vi "UMLEditor reversedEngineeringRecursiveInheritInfo.vi"(1 "localIn":T1 {"block"."bounds"."height" format="%.2f"; "block"."bounds"."width" format="%.2f"; "block"."bounds"."y" format="%.2f"; "block"."bounds"."x" format="%.2f"; "bounds"."height" format="%.2f"; "bounds"."width" format="%.2f"; "bounds"."y" format="%.2f"; "bounds"."x" format="%.2f"}, 2 "nodeIndex":i32, 3 "widthGap":i32=50, 4 "heightGap":i32=50, 5 "error in (no error)":errorcluster, 7 "allInheritorIn":i32[](array[numeric])) -> (9 "BlockHeight":i32, 11 "myHeight":i32, 13 "myWidth":i32, 14 "inheritorFound":bool, 15 "width":i32, 16 "myInheritor":i32[](array[numeric]), 17 "allInheritor":i32[](array[numeric]), 18 "myInheritorWidth":i32[](array[numeric]), 19 "error out":errorcluster)   [LabVIEW 2012]
doc: "Gets current diagram values"
uses:
  <resource>/Framework/Providers/Open_GDS/UML/UMLEditor/UMLEditor RevEngLocalvarType.ctl
  <resource>/Framework/Providers/Open_GDS/UML/Graph_class/Graph.lvclass
  <resource>/Framework/Providers/Open_GDS/UML/Graphics_class/Graphics.lvclass
  <resource>/Framework/Providers/Open_GDS/UML/Grid_class/Grid.lvclass
  <resource>/Framework/Providers/Open_GDS/UML/ClassNode_class/ClassNode.lvclass
  <resource>/Framework/Providers/Open_GDS/UML/AbstractEdge_class/AbstractEdge.lvclass
  <resource>/Framework/Providers/Open_GDS/UML/AbstractNode_class/AbstractNode.lvclass
  <resource>/Framework/Providers/Open_GDS/UML/ReversedEngineering/ReversedEngineering ClassInfoType.ctl
  <resource>/Framework/Providers/Open_GDS/UML/UMLEditor/UMLEditor_VisibilityType.ctl
  <resource>/Framework/Providers/Open_GDS/UML/ReversedEngineering/ReversedEngineering AttributeInfoType.ctl
  <resource>/Framework/Providers/Open_GDS/ClassProviders/Common/CommonVIs/CommonVIs_AttributeDataType.ctl
  <resource>/Framework/Providers/Open_GDS/UML/ReversedEngineering/ReversedEngineering_ClassDependencyDetailsType.ctl
  <resource>/Framework/Providers/Open_GDS/ClassProviders/Common/ScriptingFunctions/SubVIs/Scripting_ViDependencyType.ctl
  <resource>/Framework/Providers/Open_GDS/UML/General/Rectangle/Rectangle Rectangle2D.ctl
  <resource>/Framework/Providers/Open_GDS/UML/ReversedEngineering/ReversedEngineering TypeDefType.ctl
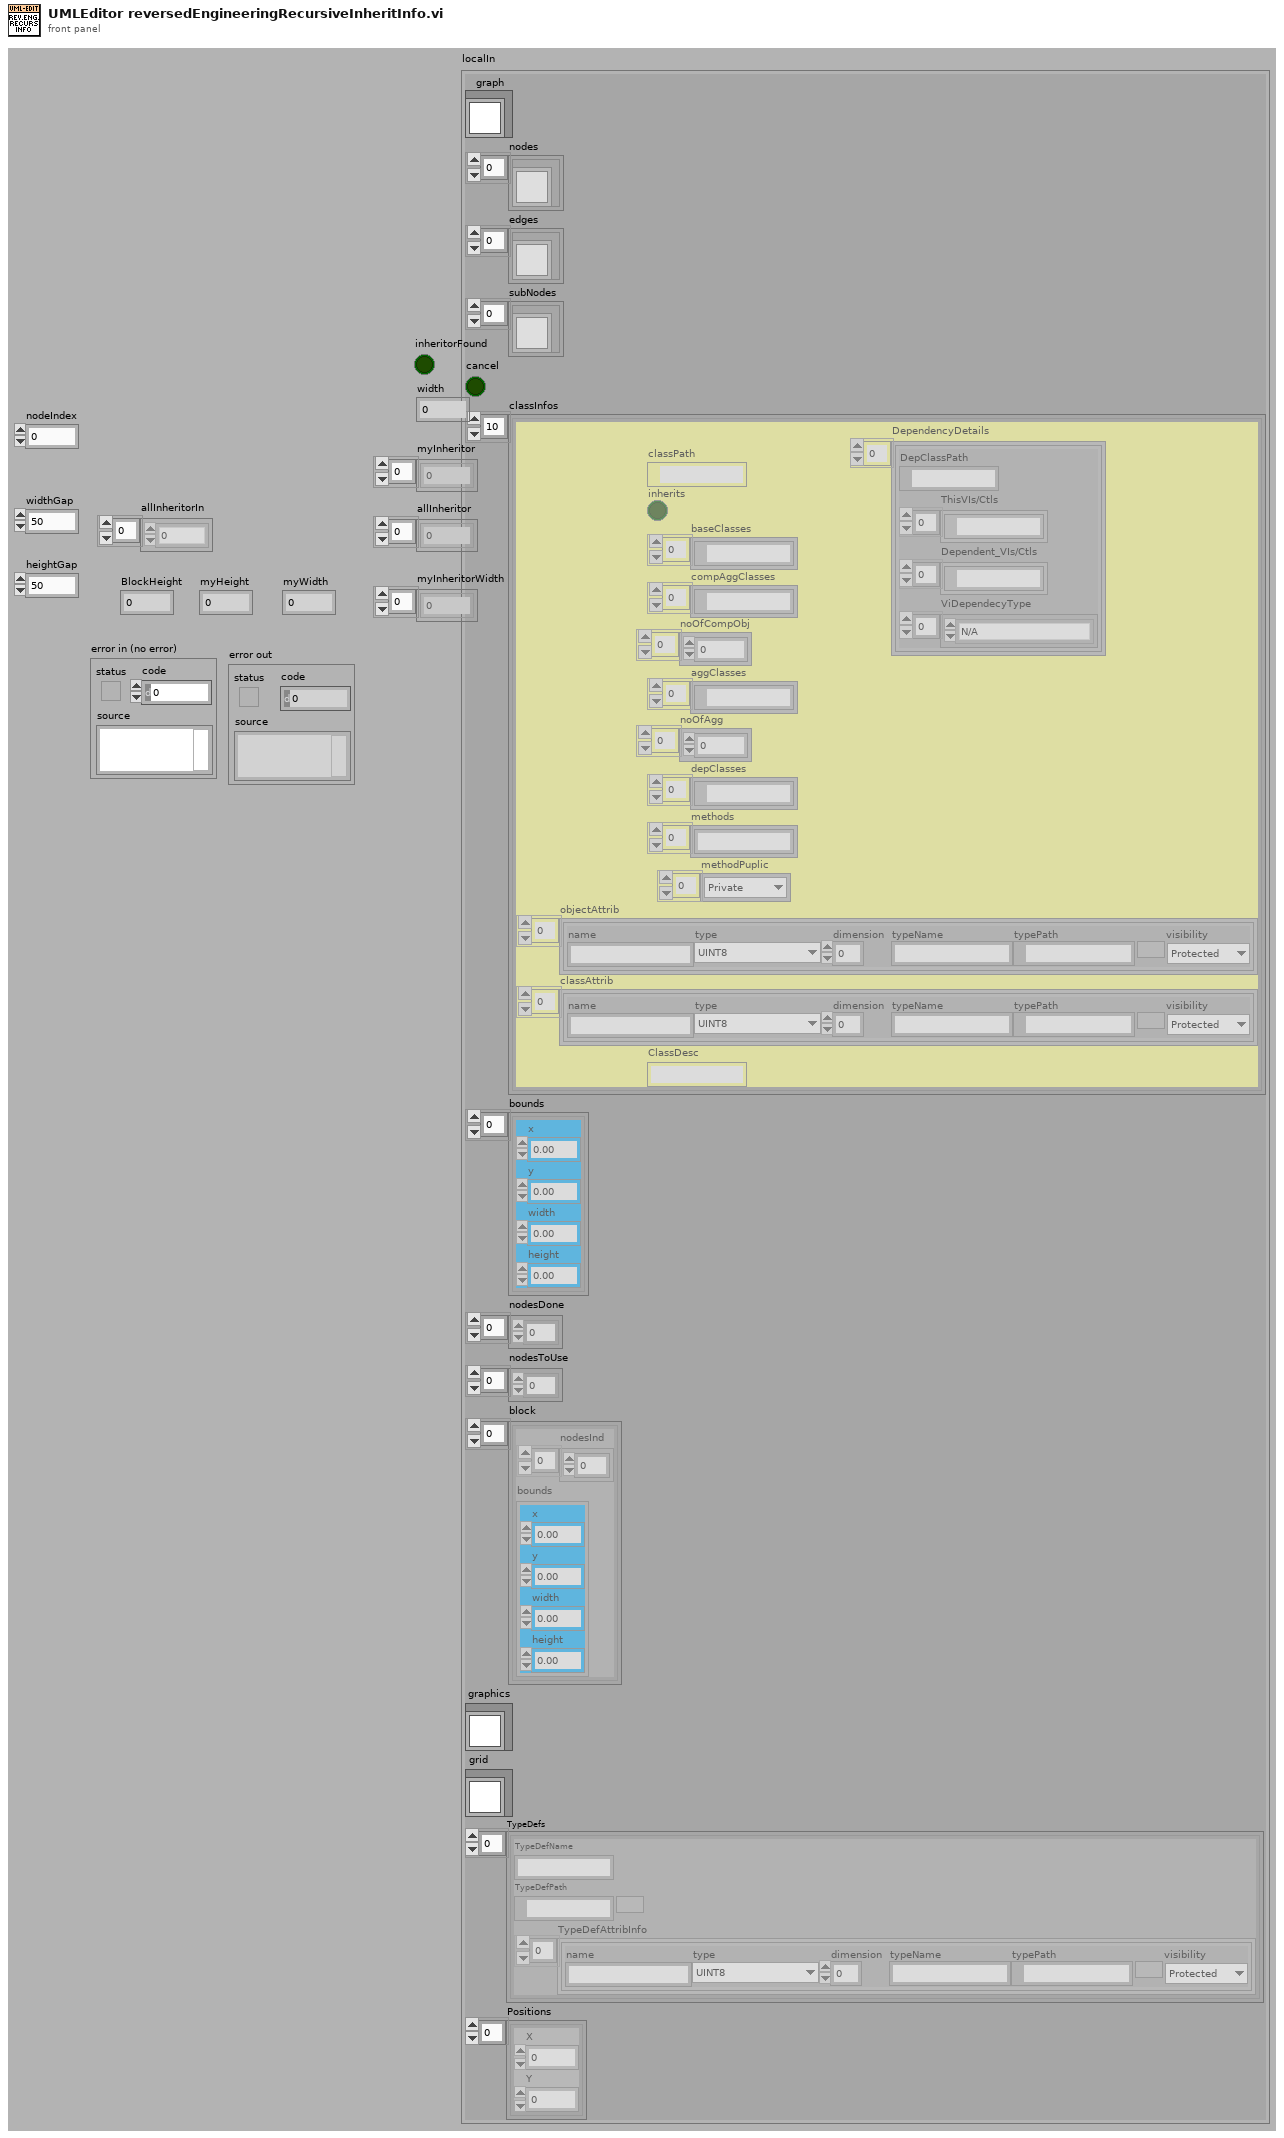
[diagram p1: front panel]
types:
  T1 = typedef "UMLEditor RevEngLocalvarType.ctl" = cluster{"graph":refnum<class "Graph.lvclass">, "nodes":refnum<class "ClassNode.lvclass">[], "edges":refnum<class "AbstractEdge.lvclass">[], "subNodes":refnum<class "AbstractNode.lvclass">[], "cancel":bool, "classInfos":T2[], "bounds":T8[], "nodesDone":i32[], "nodesToUse":i32[], "block":cluster{"nodesInd":i32[], "bounds":T8}[], "graphics":refnum<class "Graphics.lvclass">, "grid":refnum<class "Grid.lvclass">, "TypeDefs":T9[], "Positions":cluster{"X":i32, "Y":i32}[]}
  T2 = typedef "ReversedEngineering ClassInfoType.ctl" = cluster{"classPath":path, "inherits":bool, "baseClasses":path[], "compAggClasses":path[], "noOfCompObj":i32[], "aggClasses":path[], "noOfAgg":i32[], "depClasses":path[], "methods":string[], "methodPuplic":T3[], "objectAttrib":T4[], "classAttrib":T4[], "ClassDesc":string, "DependencyDetails":T6[]}
  T3 = typedef "UMLEditor_VisibilityType.ctl" = enum16{"Public", "Private", "Protected"}
  T4 = typedef "ReversedEngineering AttributeInfoType.ctl" = cluster{"name":string, "type":T5, "dimension":i32, "typeName":string, "typePath":path, "visibility":T3}
  T5 = typedef "CommonVIs_AttributeDataType.ctl" = enum16{"UINT8", "INT8", "UINT16", "INT16", "UINT32", "INT32", "UINT64", "INT64", "SGL", "DBL", "EXT", "CSG", "CDB", "CXT", "TimeStamp", "STRING", "PATH", "BOOL", "ENUM", "RefNum", "VIRefNum", "LabVIEW Class", "Cluster", "Variant", "TypeDef", "Waveform", "LabVIEW Object", "Other", "void"}
  T6 = typedef "ReversedEngineering_ClassDependencyDetailsType.ctl" = cluster{"DepClassPath":path, "ThisVIs/Ctls":path[], "Dependent_VIs/Ctls":path[], "ViDependecyType":T7[]}
  T7 = typedef "Scripting_ViDependencyType.ctl" = enum16{"N/A", "Launches"}
  T8 = typedef "Rectangle Rectangle2D.ctl" = cluster{"x":dbl, "y":dbl, "width":dbl, "height":dbl}
  T9 = typedef "ReversedEngineering TypeDefType.ctl" = cluster{"TypeDefName":string, "TypeDefPath":path, "TypeDefAttribInfo":T4[]}
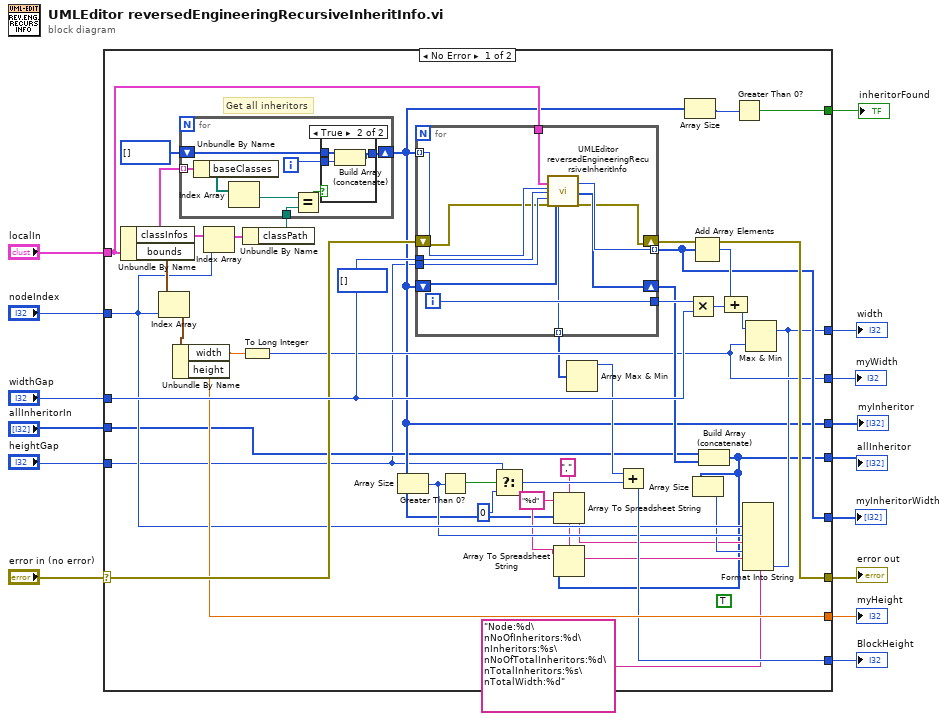
[diagram p0: block diagram]
diagram:
  n1 = case shown="No Error" "error in (no error)" {
    selector: "error in (no error)" -> [w43 w79]
    tunnel: [w42 w79] -> w14
    tunnel: "localIn" -> [w49 _]
    tunnel: "nodeIndex" -> [w26 _]
    tunnel: "widthGap" -> [w47 _]
    tunnel: [w27 _] -> w10
    tunnel: [w19 _] -> w9
    tunnel: [w18 _] -> w8
    tunnel: [w39 _] -> w7
    tunnel: [w38 _] -> w6
    tunnel: [w36 _] -> w5
    tunnel: [w35 _] -> w4
    tunnel: "heightGap" -> [w16 _]
    tunnel: [w31 _] -> w2
    tunnel: "allInheritorIn" -> [w17 _]
    frame No Error {
      (unwired) i32[] []
      w22 = "%d" ("format string")
      (unwired) TRUE ("convert eol? (no:F)")
      w21 = "," ("delimiter (Tab)")
      # "Get all inheritors"
      n2 = Unbundle By Name(w49) -> ("classInfos"=w52:T2[], "bounds"=w53:T8[])
      n3 = Index Array(array=w53, index=w26) -> (element=w55:T8)
      n4 = Unbundle By Name(w55) -> ("width"=w46:dbl, "height"=w35:dbl)
      n5 = Index Array(array=w52, index=w26) -> (element=w54:T2)
      n6 = To Long Integer(number=w46) -> (32bit integer=w38:i32)
      n7 = Unbundle By Name(w54) -> ("classPath"=w51:path)
      n8 = for {
        tunnel: w52 -> [w74] mode=indexing
        shift-right: [w68] -> w18
        shift-left: i32[] [] -> [w69]
        tunnel: w51 -> [w71]
        i -> [w67]
        n9 = Unbundle By Name(w74) -> ("baseClasses"=w73:path[])
        n10 = Index Array(array=w73) -> (element=w72:path)  [unwired: 1 in]
        n11 = Equal?(x=w72, y=w71) -> (x = y?=w70:bool)
        n12 = case shown="True" w70 {
          tunnel: w69 -> [w75 w78]
          tunnel: [w75 w77] -> w68
          tunnel: w67 -> [_ w76]
          frame False {
          }
          frame True {
            n13 = Build Array (concatenate)(w78, w76) -> (w77:i32[])
          }
        }
      }
      n14 = Array Size(array=w18) -> (size(s)=w25:i32)
      n15 = for {
        tunnel: w18 -> [w61] mode=indexing
        tunnel: w49 -> [w65]
        tunnel: w47 -> [w60]
        tunnel: [w64] -> w39 mode=indexing
        tunnel: [w66] -> w48
        shift-right: [w62] -> w42
        shift-left: w43 -> [w58]
        shift-right: [w63] -> w40
        shift-left: w18 -> [w57]
        tunnel: [w56] -> w30 mode=indexing
        tunnel: w16 -> [w59]
        i -> [w66]
        n16 = call <resource>:"UMLEditor reversedEngineeringRecursiveInheritInfo.vi"("localIn"=w65, "nodeIndex"=w61, "widthGap"=w60, "heightGap"=w59, "error in (no error)"=w58, "allInheritorIn"=w57) -> ("BlockHeight"=w56:i32, "width"=w64:i32, "allInheritor"=w63:i32[], "error out"=w62:errorcluster)  [unwired: 5 in, 5 out]
      }
      n17 = Greater Than 0?(x=w25) -> (x > 0?=w34:bool)
      n18 = Select(t=w16, s=w34, f=0) -> (s? t:f=w32:i32)
      n19 = Array To Spreadsheet String(delimiter (Tab)=w21, array=w18, 3:w22) -> (spreadsheet string=w23:string)
      n20 = Array Max & Min(array=w30) -> (max value=w29:i32)  [unwired: 3 out]
      n21 = Add(x=w29, y=w32) -> (x+y=w31:i32)
      n22 = Array Size(array=w18) -> (size(s)=w37:i32)
      n23 = Multiply(x=w48, y=w47) -> (x*y=w45:i32)
      n24 = Add Array Elements(numeric array=w39) -> (sum=w44:i32)
      n25 = Build Array (concatenate)(w17, w40) -> (w19:i32[])
      n26 = Array To Spreadsheet String(delimiter (Tab)=w21, array=w19, 3:w22) -> (spreadsheet string=w20:string)
      n27 = Array Size(array=w19) -> (size(s)=w24:i32)
      n28 = Compound Arithmetic op=ADD(w44, w45) -> (w41:i32)
      n29 = Greater Than 0?(x=w37) -> (x > 0?=w36:bool)
      n30 = Max & Min(x=w41, y=w38) -> (max(x,y)=w27:i32)  [unwired: 1 out]
      n31 = Format Into String(format string="Node:%d\nNoOfInheritors:%d\nInheritors:%s\nNoOfTotalInheritors:%d\nTotalInheritors:%s\nTotalWidth:%d", w26, w25, w23, w24, w20, w27) -> ()  [unwired: 2 in, 2 out]
    }
    frame Error {
    }
  }
  "error out" <- w14
  "width" <- w10
  "allInheritor" <- w9
  "myInheritor" <- w8
  "myInheritorWidth" <- w7
  "myWidth" <- w6
  "inheritorFound" <- w5
  "myHeight" <- w4
  "BlockHeight" <- w2
